vi "select energy_old.vi"(8 "Error In":errorcluster, 9 "List ROI in":dbl[][](array[numeric]), 10 "List Peak":string[][](table)=[["0", "0.738169", "8216.078017"], ["1", "1.925791", "11797.605609"], ["2", "2.296686", "59445.586632"], ["3", "2.951953", "7958.809520"], ["4", "3.301930", "5536.954047"], ["5", "3.693063", "592063.911968"], ["6", "4.012579", "88599.650063"], ["7", "5.456304", "6013.116723"], ["8", "5.905392", "7038.874622"], ["9", "6.404196", "22471.618393"], ["10", "7.049745", "8038.961303"], ["11", "7.336853", "5649.863203"], ["12", "7.978842", "3458.992769"], ["13", "8.617482", "7301.160509"], ["14", "9.554502", "1097.160220"], ["15", "10.523191", "20487.327187"], ["16", "11.054270", "2935.510385"], ["17", "11.234771", "2776.270069"], ["18", "12.573155", "28067.247871"], ["19", "13.048495", "7100.524309"], ["20", "13.060056", "7093.993228"], ["21", "13.100857", "7126.608473"], ["22", "13.283153", "7227.068614"], ["23", "14.060270", "10970.472713"], ["24", "14.659482", "8813.189447"], ["25", "15.701110", "4886.263831"], ["26", "16.589220", "151655.425908"], ["27", "17.295466", "73726.613413"], ["28", "18.547307", "16625.597400"], ["29", "19.386897", "11325.808412"], ["30", "23.791659", "1504.095156"], ["31", "24.239552", "1887.308691"], ["32", "24.942128", "13678.898904"]], 11 "Spectrum":cluster{"Channels":dbl[], "Intensity":dbl[]}[](graph)) -> (0 "Error Out":errorcluster, 1 "List ROI in out":dbl[][](array[numeric]), 2 "Peak Position":cluster{"Array":dbl[], "Array":dbl[]}, 3 "Elements":string[][](table))   [LabVIEW 2020]
uses:
  <vilib>/Utility/miscctls.llb/LVRowAndColumnTypeDef.ctl
  e287f4bb-419c-b64e-b283-fdec1ab58d66.vi
  8e2a2df9-f711-f049-943d-4995b6f05a7b.vi
  95577ca1-b70a-e540-a978-da85c0e4bb45.vi
  <vilib>/Utility/Data Type/Get Array Information.vi
  <vilib>/Utility/Data Type/Get Type Information.vi
panel:
  in  "Add":bool
  in  "ordinate":u16(ring) items=["Linear", "Logarithmic"]
  in  "doubt":bool
  in  "reset":bool
  out "List In":cluster{"Channels":dbl[], "Intensity":dbl[]}
  out "Data In":cluster{"Channels":dbl[], "Intensity":dbl[]}
  out "Element Position Peaks":dbl[][](array[numeric])
  out "Best Match":string[][](table)
  in  "exit":bool
  # "?"
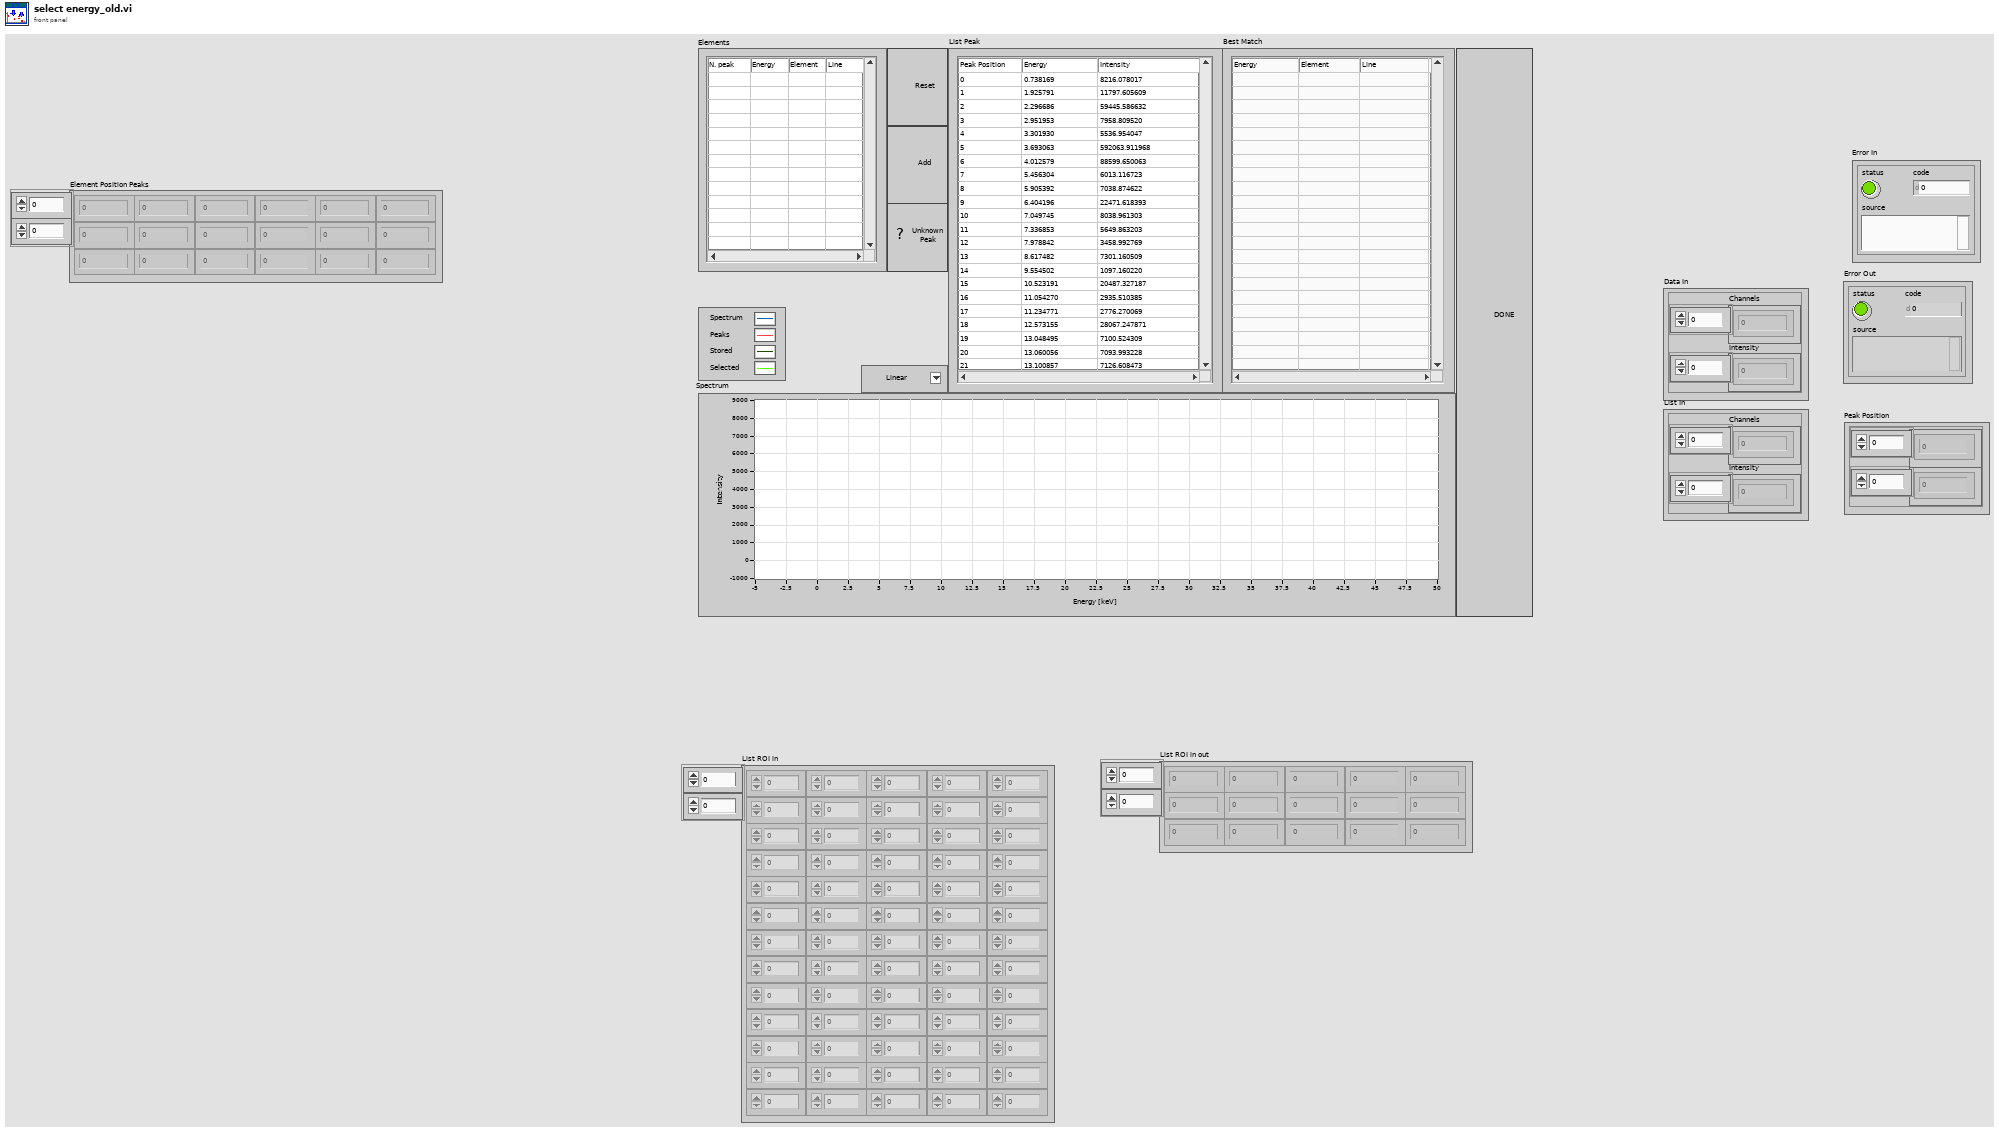
[diagram p1: front panel]
types:
  T1 = typedef "LVRowAndColumnTypeDef.ctl" = cluster{"Row":i32, "Column":i32}
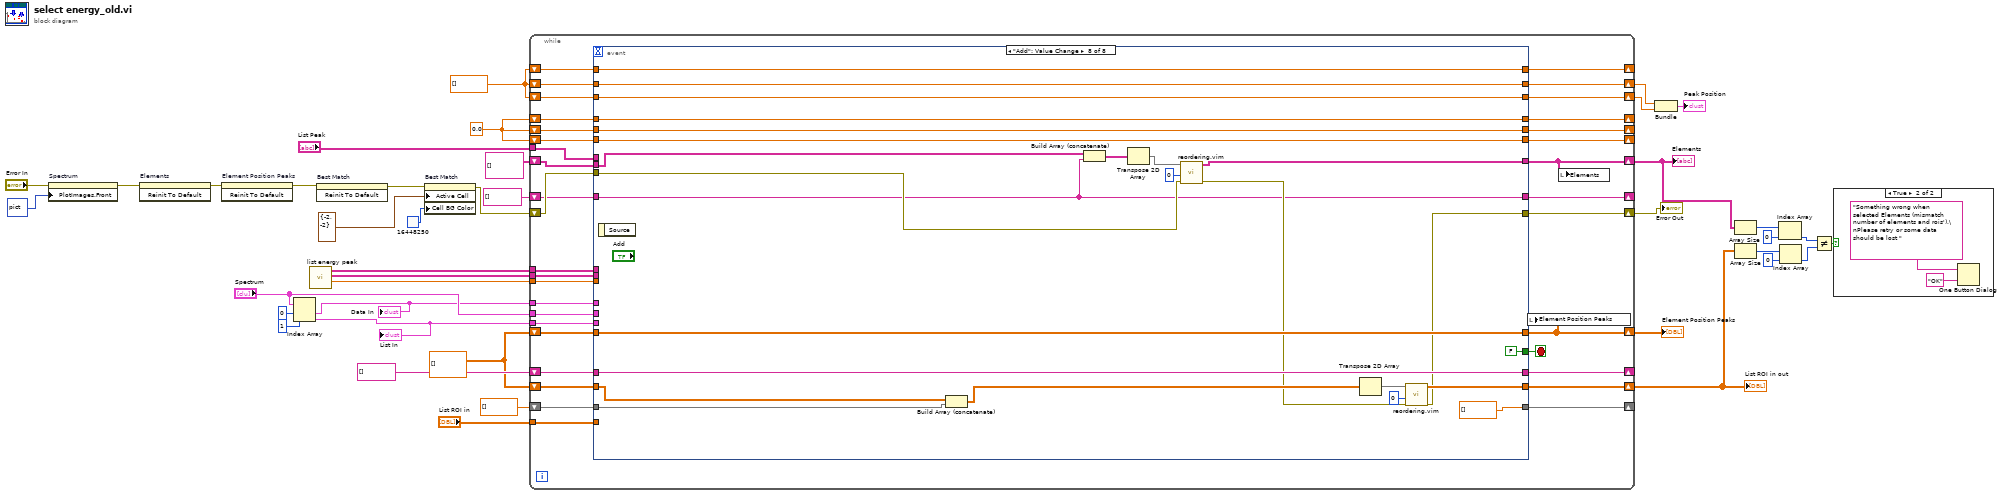
[diagram p0: block diagram]
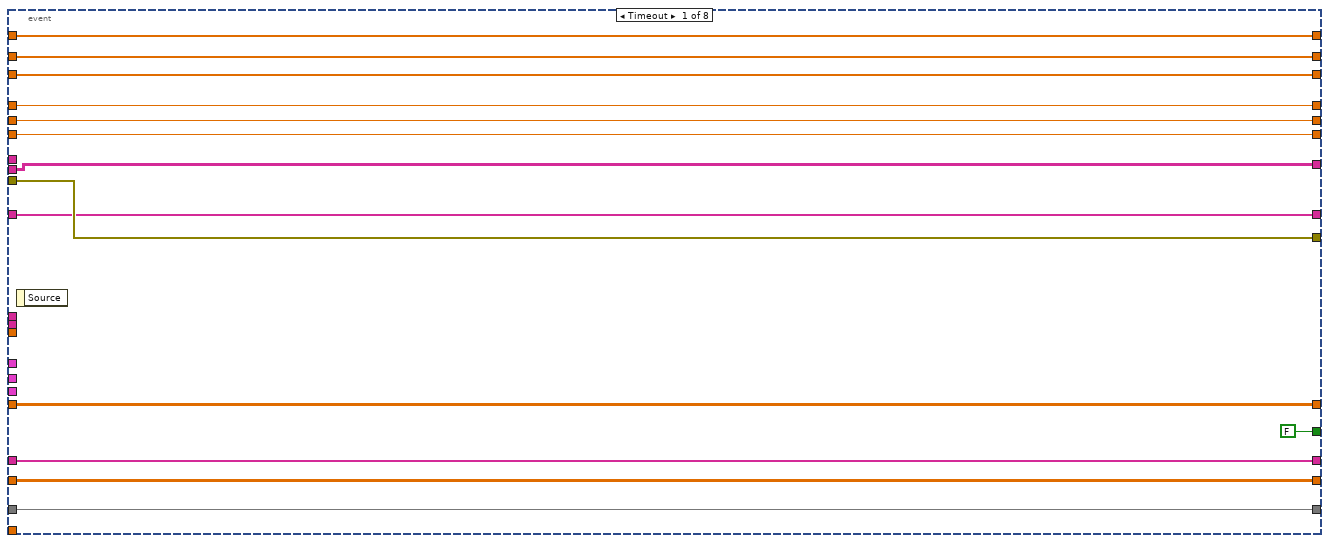
[diagram p3: hidden frame]
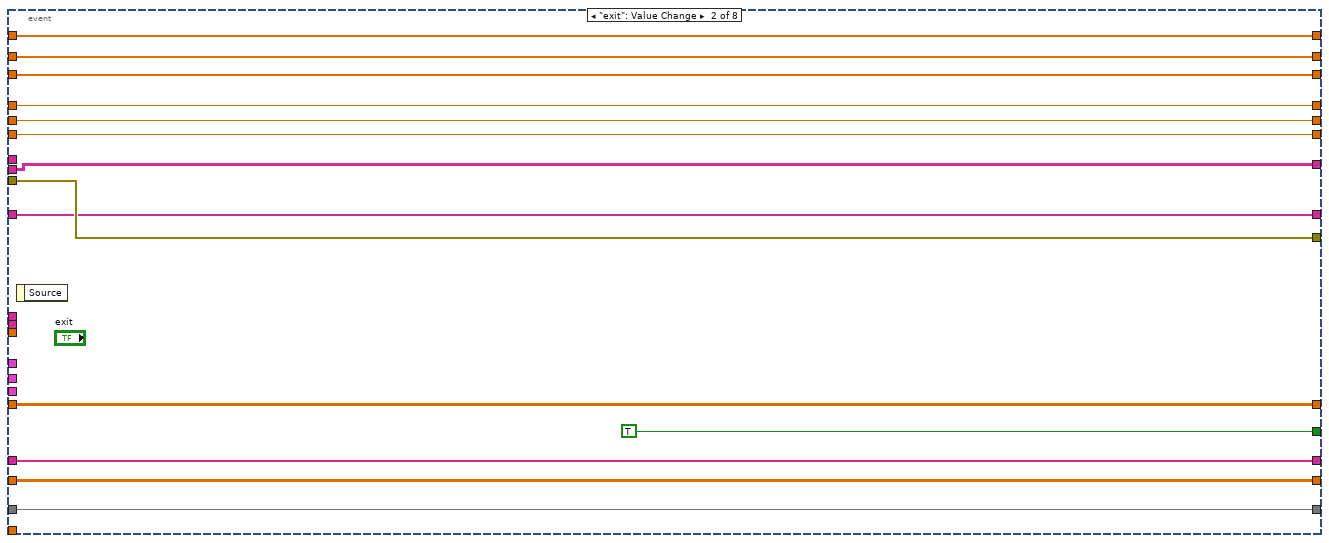
[diagram p4: hidden frame]
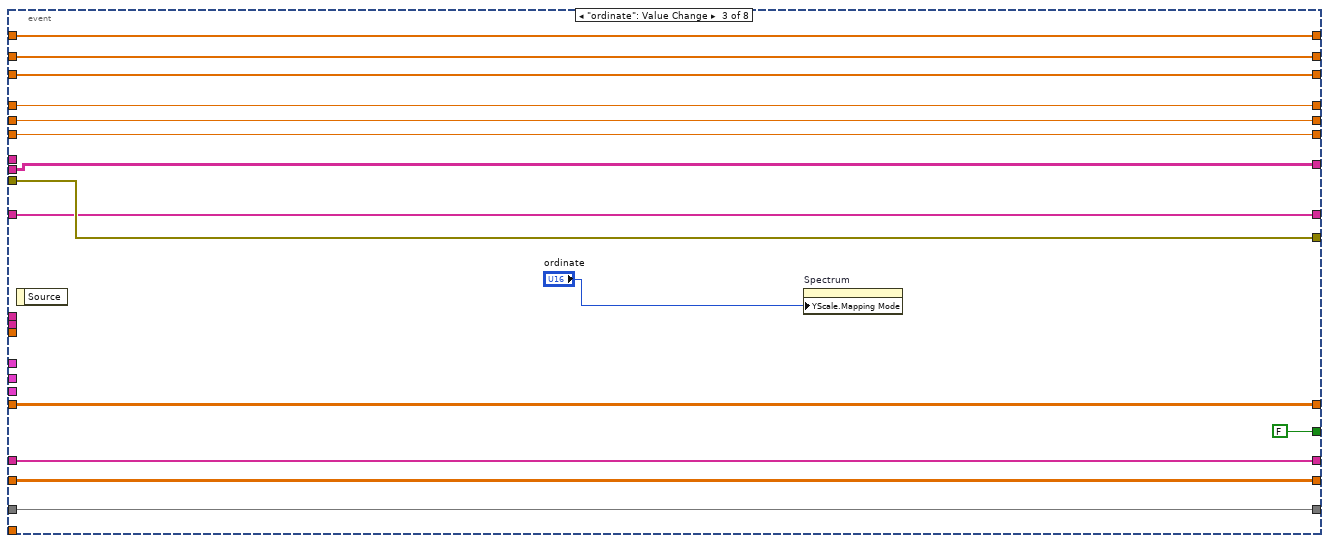
[diagram p5: hidden frame]
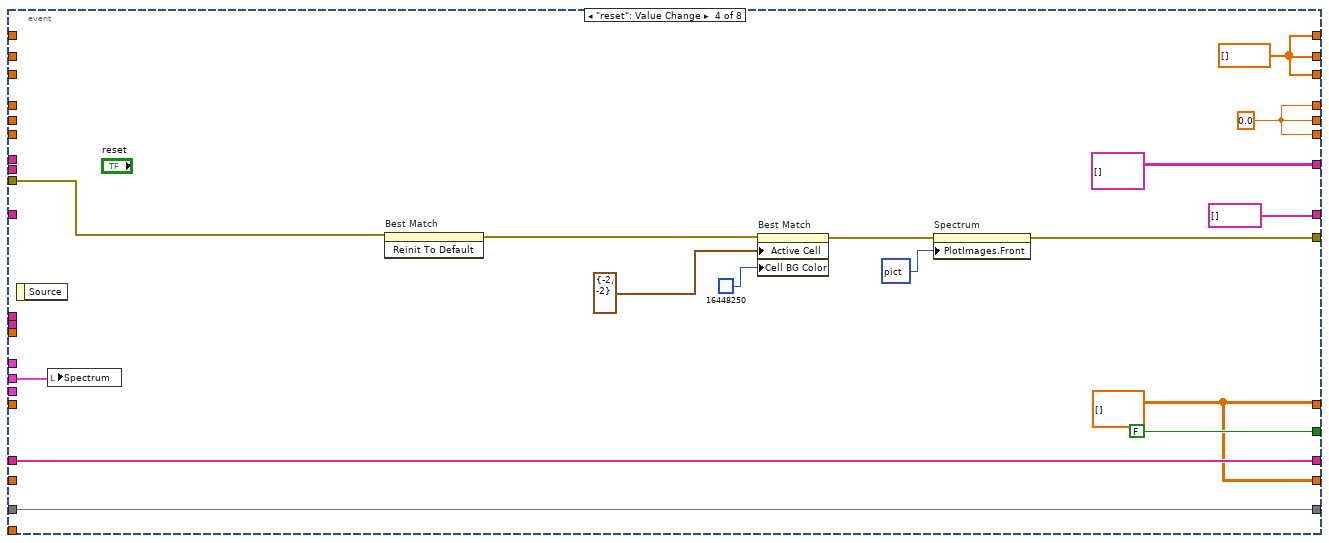
[diagram p6: hidden frame]
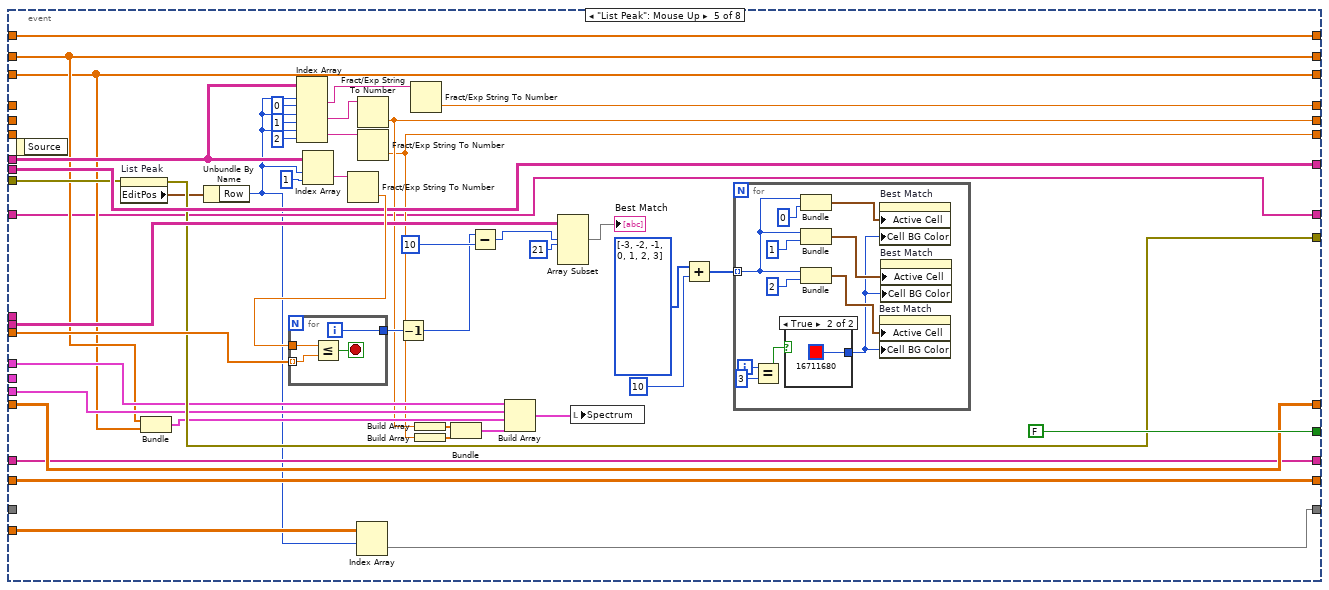
[diagram p7: hidden frame]
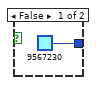
[diagram p8: hidden frame]
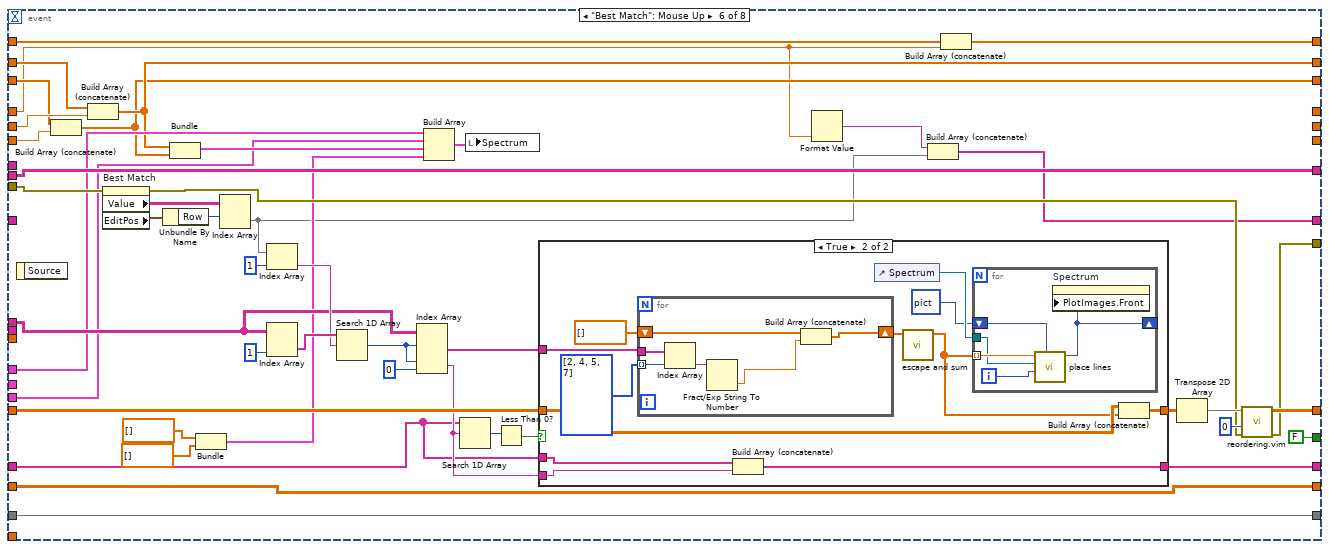
[diagram p9: hidden frame]
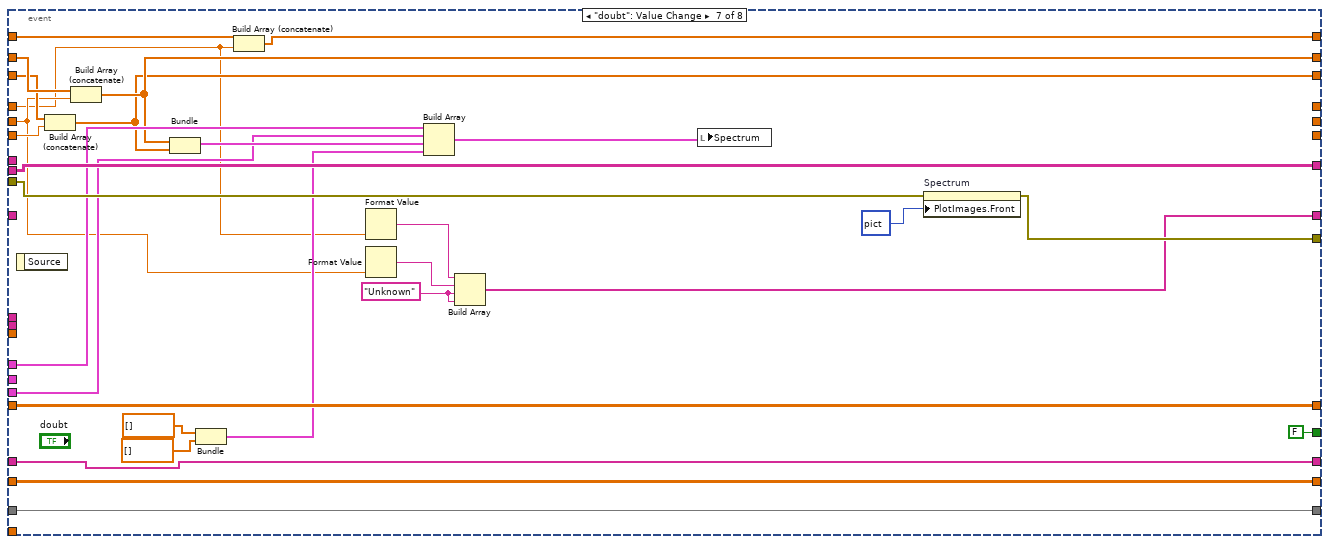
[diagram p11: hidden frame]
diagram:
  w2 = 0.0
  w1 = dbl[] []
  w13 = dbl[][] []
  n1 = property on="Spectrum" class="XYGraph (strict)"(error in="Error In", "PlotImages.Front"=picture data[5B] ("line to place")) -> (error out=w25:errorcluster)  [unwired: 1 in, 1 out]
  n2 = invoke on="Elements" class="Tbl (strict)" method="Reinit To Default"(error in=w25) -> (error out=w31:errorcluster)  [unwired: 2 in, 2 out]
  n3 = invoke on="Element Position Peaks" class="Arr (strict)" method="Reinit To Default"(error in=w31) -> (error out=w30:errorcluster)  [unwired: 2 in, 2 out]
  n4 = Index Array(array="Spectrum", index #1=0 ("index"), index #2=1 ("index")) -> (element #1=w20:cluster{"Channels":dbl[], "Intensity":dbl[]}, element #2=w19:cluster{"Channels":dbl[], "Intensity":dbl[]})
  "Data In" <- w20
  "List In" <- w19
  n5 = call "list energy peak.vi"() -> ("Energies Ordered"=w39:dbl[], "List Ordered"=w40:string[][], "List"=w34:string[][])  [unwired: 9 in]
  n6 = invoke on="Best Match" class="Tbl (strict)" method="Reinit To Default"(error in=w30) -> (error out=w37:errorcluster)  [unwired: 2 in, 2 out]
  n7 = property on="Best Match" class="Tbl (strict)"(error in=w37, "Active Cell"=T1 {"Row"=-2, "Column"=-2} ("Active Cell:Active Cell"), "Cell BG Color"=u32 16448250) -> (error out=w29:errorcluster)  [unwired: 1 in, 1 out]
  n8 = while {
    tunnel: "List Peak" -> [w75]
    tunnel: w40 -> [w72]
    tunnel: w39 -> [w74]
    tunnel: w34 -> [w71]
    shift-right: [w68] -> w7
    shift-left: string[][] [] -> [w70]
    shift-right: [w67] -> w32
    shift-left: w13 -> [w69]
    tunnel: "Spectrum" -> [w60]
    shift-right: [w66] -> w28
    shift-left: w29 -> [w65]
    shift-right: [w64] -> _
    shift-left: string[] [] -> [w63]
    shift-right: [w62] -> w17
    shift-left: w1 -> [w61]
    shift-right: [w59] -> w18
    shift-left: w1 -> [w58]
    tunnel: w20 -> [w57]
    tunnel: w19 -> [w56]
    shift-right: [w54] -> _
    shift-left: w2 -> [w52]
    shift-right: [w55] -> _
    shift-left: w2 -> [w53]
    shift-right: [w51] -> _
    shift-left: string[] [] ("Value") -> [w50]
    shift-right: [w49] -> w6
    shift-left: w13 -> [w48]
    tunnel: "List ROI in" -> [w47]
    shift-right: [w45] -> _
    shift-left: dbl[] [] -> [w46]
    shift-right: [w44] -> _
    shift-left: w2 -> [w43]
    shift-right: [w42] -> _
    shift-left: w1 -> [w41]
    stop <- w73 stop-if-true
    n9 = event shown="[7] \"Add\": Value Change" {
      selector: _ -> [_ _ _ _ _ _ _ _]
      dyn-events: _ -> [_ _ _ _ _ _ _ _]
      timeout: _ -> [_ _ _ _ _ _ _ _]
      tunnel: w75 -> [_ _ _ _ w159 _ _ _]
      tunnel: w74 -> [_ _ _ _ w177 _ _ _]
      tunnel: [FALSE ("Stop Button") TRUE ("Stop Button") FALSE ("Stop Button") FALSE ("Stop Button") FALSE ("Stop Button") FALSE ("Stop Button") FALSE ("Stop Button") FALSE ("Stop Button")] -> w73
      tunnel: w72 -> [_ _ _ _ w174 _ _ _]
      tunnel: w71 -> [_ _ _ _ _ w237 _ _]
      tunnel: [w88 w102 w117 string[][] [] ("Data Out") w165 w236 w298 w315] -> w68
      tunnel: w70 -> [w88 w102 w117 _ w165 w236 w298 w316]
      tunnel: [w87 w101 w116 w121 w164 w233 w297 w312] -> w67
      tunnel: w69 -> [w87 w101 w116 _ w164 w235 w297 w312]
      tunnel: [w86 w100 w115 w125 w162 w227 w280 w303] -> w66
      tunnel: w65 -> [w86 w100 w115 w129 w163 w229 w295 w314]
      tunnel: [w85 w99 w114 w128 w161 w221 w282 w311] -> w64
      tunnel: w63 -> [w85 w99 w114 w128 w161 w220 w282 w311]
      tunnel: [w84 w97 w112 w119 w150 w207 w283 w322] -> w62
      tunnel: w61 -> [w84 w97 w112 _ w150 w209 w285 w322]
      tunnel: w60 -> [_ _ _ w124 _ _ _ _]
      tunnel: [w83 w98 w113 w119 w151 w210 w286 w323] -> w59
      tunnel: w58 -> [w83 w98 w113 _ w151 w212 w287 w323]
      tunnel: w57 -> [_ _ _ _ w153 w217 w292 _]
      tunnel: w56 -> [_ _ _ _ w152 w216 w291 _]
      tunnel: [w82 w96 w111 w120 w145 _ _ w321] -> w55
      tunnel: [w81 w95 w110 w120 w144 _ _ w320] -> w54
      tunnel: w53 -> [w82 w96 w111 _ _ w211 w273 w321]
      tunnel: w52 -> [w81 w95 w110 _ _ w208 w284 w320]
      tunnel: [w80 w94 w108 string[] [] ("Value") w143 w199 w277 w299] -> w51
      tunnel: w50 -> [w80 w94 w108 _ w143 _ _ w299]
      tunnel: [w79 w93 w107 w121 w142 w204 w275 w305] -> w49
      tunnel: w48 -> [w79 w93 w107 _ w142 w204 w275 w310]
      tunnel: w47 -> [_ _ _ _ w141 _ _ _]
      tunnel: w46 -> [w78 w92 w106 w122 _ w205 w276 w309]
      tunnel: [w78 w92 w106 w122 w140 w205 w276 dbl[] []] -> w45
      tunnel: [w77 w91 w105 w120 w136 _ _ w301] -> w44
      tunnel: w43 -> [w77 w91 w105 _ _ w201 w270 w301]
      tunnel: [w76 w90 w104 w119 w135 w202 w272 w300] -> w42
      tunnel: w41 -> [w76 w90 w104 _ w135 w203 w274 w300]
      event Timeout {
        n10 = event-data() -> ()  [unwired: 1 in, 1 out]
      }
      event "exit": Value Change {
        n11 = event-data() -> ()  [unwired: 1 in, 1 out]
      }
      event "ordinate": Value Change {
        n12 = event-data() -> ()  [unwired: 1 in, 1 out]
        n13 = property on="Spectrum" class="XYGraph (strict)"("YScale.Mapping Mode"="ordinate") -> ()  [unwired: 2 in, 2 out]
      }
      event "reset": Value Change {
        w120 = 0.0
        w119 = dbl[] []
        w121 = dbl[][] [] ("Data Out")
        n14 = event-data() -> ()  [unwired: 1 in, 1 out]
        n15 = local write "Spectrum"(w124) -> ()
        n16 = invoke on="Best Match" class="Tbl (strict)" method="Reinit To Default"(error in=w129) -> (error out=w134:errorcluster)  [unwired: 2 in, 2 out]
        n17 = property on="Best Match" class="Tbl (strict)"(error in=w134, "Active Cell"=T1 {"Row"=-2, "Column"=-2} ("Active Cell:Active Cell"), "Cell BG Color"=u32 16448250) -> (error out=w126:errorcluster)  [unwired: 1 in, 1 out]
        n18 = property on="Spectrum" class="XYGraph (strict)"(error in=w126, "PlotImages.Front"=picture data[5B] ("line to place")) -> (error out=w125:errorcluster)  [unwired: 1 in, 1 out]
      }
      event "List Peak": Mouse Up {
        n19 = event-data() -> ()  [unwired: 1 in, 1 out]
        n20 = property on="List Peak" class="Tbl (strict)"(error in=w163) -> (error out=w162:errorcluster, "EditPos"=w160:T1)  [unwired: 1 in, 1 out]
        n21 = Bundle(w151, w150) -> (w149:cluster{dbl[], dbl[]})  [unwired: 1 in]
        n22 = Unbundle By Name(w160) -> ("Row"=w139:i32)
        n23 = Index Array(array=w159, index (row) #1=w139, index (col) #1=0 ("disabled index (col)"), index (row) #2=w139, index (col) #2=1 ("disabled index (col)"), index (row) #3=w139, index (col) #3=2 ("disabled index (col)")) -> (element #1=w137:string, element #2=w156:string, element #3=w155:string)
        n24 = Index Array(array=w159, index (row)=w139, index (col)=1 ("disabled index (col)")) -> (element=w179:string)
        n25 = Fract/Exp String To Number(string=w179) -> (number=w178:dbl)  [unwired: 3 in, 1 out]
        n26 = for {
          tunnel: w178 -> [w197]
          tunnel: w177 -> [w196] mode=indexing
          tunnel: [w194] -> w175
          i -> [w194]
          stop <- w195 stop-if-true
          n27 = Less Or Equal?(x=w197, y=w196) -> (x <= y?=w195:bool)
        }
        n28 = Index Array(array=w141, index (row)=w139) -> (element=w140:dbl[])  [unwired: 1 in]
        n29 = Fract/Exp String To Number(string=w156) -> (number=w145:dbl)  [unwired: 3 in, 1 out]
        n30 = Fract/Exp String To Number(string=w155) -> (number=w144:dbl)  [unwired: 3 in, 1 out]
        n31 = Decrement(x=w175) -> (x-1=w168:i32)
        n32 = Fract/Exp String To Number(string=w137) -> (number=w136:dbl)  [unwired: 3 in, 1 out]
        n33 = Build Array(w145) -> (w147:dbl[])
        n34 = Build Array(w144) -> (w146:dbl[])
        n35 = Bundle(w147, w146) -> (w148:cluster{dbl[], dbl[]})  [unwired: 1 in]
        n36 = Subtract(x=w168, y=10) -> (x-y=w171:i32)
        n37 = Build Array(w153, w152, w149, w148) -> (w154:cluster{"Channels":dbl[], "Intensity":dbl[]}[])
        n38 = Array Subset(array=w174, index (row)=w171, length (row)=21 ("length")) -> (→"Best Match":string[][])  [unwired: 2 in]
        n39 = local write "Spectrum"(w154) -> ()
        n40 = Add(x=i32[] [-3, -2, -1, 0, 1, 2, 3], y=10) -> (x+y=w167:i32[])
        n41 = for {
          tunnel: w167 -> [w183] mode=indexing
          i -> [w191]
          n42 = Equal?(x=w191, y=3) -> (x = y?=w189:bool)
          n43 = case shown="True" w189 {
            tunnel: [u32 9567230 u32 16711680] -> w181
            frame False {
            }
            frame True {
            }
          }
          n44 = Bundle(w183, 0) -> (w182:cluster{i32, i32})  [unwired: 1 in]
          n45 = Bundle(w183, 1) -> (w186:cluster{i32, i32})  [unwired: 1 in]
          n46 = Bundle(w183, 2) -> (w185:cluster{i32, i32})  [unwired: 1 in]
          n47 = property on="Best Match" class="Tbl (strict)"("Active Cell"=w182, "Cell BG Color"=w181) -> ()  [unwired: 2 in, 2 out]
          n48 = property on="Best Match" class="Tbl (strict)"("Active Cell"=w185, "Cell BG Color"=w181) -> ()  [unwired: 2 in, 2 out]
          n49 = property on="Best Match" class="Tbl (strict)"("Active Cell"=w186, "Cell BG Color"=w181) -> ()  [unwired: 2 in, 2 out]
        }
      }
      event "Best Match": Mouse Up {
        n50 = event-data() -> ()  [unwired: 1 in, 1 out]
        n51 = Build Array (concatenate)(w209, w208) -> (w207:dbl[])
        n52 = Build Array (concatenate)(w212, w211) -> (w210:dbl[])
        n53 = property on="Best Match" class="Tbl (strict)"(error in=w229) -> (error out=w228:errorcluster, "Value"=w243:string[][], "EditPos"=w244:T1)  [unwired: 1 in, 1 out]
        n54 = Unbundle By Name(w244) -> ("Row"=w206:i32)
        n55 = Bundle(w210, w207) -> (w218:cluster{dbl[], dbl[]})  [unwired: 1 in]
        n56 = Bundle(dbl[] [], dbl[] []) -> (w213:cluster{dbl[], dbl[]})  [unwired: 1 in]
        n57 = Index Array(array=w243, index (row)=w206) -> (element=w200:string[])  [unwired: 1 in]
        n58 = Index Array(array=w200, index=1) -> (element=w239:string)
        n59 = Index Array(array=w237, index (col)=1 ("disabled index (col)")) -> (element=w240:string[])  [unwired: 1 in]
        n60 = Search 1D Array(1D array=w240, element=w239) -> (index of element=w226:i32)  [unwired: 1 in]
        n61 = Index Array(array=w237, index (row) #1=w226, index (row) #2=w226, index (col) #2=0 ("disabled index (col)")) -> (element #1=w238:string[], element #2=w222:string)  [unwired: 1 in]
        n62 = Build Array(w217, w216, w218, w213) -> (w219:cluster{"Channels":dbl[], "Intensity":dbl[]}[])
        n63 = Search 1D Array(1D array=w220, element=w222) -> (index of element=w224:i32)  [unwired: 1 in]
        n64 = local write "Spectrum"(w219) -> ()
        n65 = Less Than 0?(x=w224) -> (x < 0?=w223:bool)
        n66 = case shown="True" w223 {
          tunnel: w238 -> [_ w258]
          tunnel: w235 -> [w246 w255]
          tunnel: [w246 w254] -> w232
          tunnel: w222 -> [_ w252]
          tunnel: [w245 w251] -> w221
          tunnel: w220 -> [w245 w250]
          frame False {
          }
          frame True {
            n67 = for {
              tunnel: w258 -> [w269]
              tunnel: i32[] [2, 4, 5, 7] -> [w268] mode=indexing
              shift-right: [w267] -> w253
              shift-left: dbl[] [] -> [w266]
              n68 = Index Array(array=w269, index=w268) -> (element=w265:string)
              n69 = Fract/Exp String To Number(string=w265) -> (number=w264:dbl)  [unwired: 3 in, 1 out]
              n70 = Build Array (concatenate)(w266, w264) -> (w267:dbl[])
            }
            n71 = Build Array (concatenate)(w250, w252) -> (w251:string[])
            n72 = control-ref of="Spectrum"() -> (w248:refnum<vi>)
            n73 = call "escape and sum.vi"("List in"=w253) -> ("List Out"=w249:dbl[])  [unwired: 10 in]
            n74 = for {
              tunnel: w249 -> [w263] mode=indexing
              tunnel: w248 -> [w261]
              shift-right: [w260] -> _
              shift-left: picture data[5B] ("line to place") -> [w259]
              i -> [w262]
              n75 = call "place lines.vi"("picture in"=w259, "line"=w262, "Graph"=w261, "Energy"=w263) -> ("line to place"=w260:picture)  [unwired: 7 in]
              n76 = property on="Spectrum" class="XYGraph (strict)"("PlotImages.Front"=w260) -> ()  [unwired: 2 in, 2 out]
            }
            n77 = Build Array (concatenate)(w255, w249) -> (w254:dbl[][])
          }
        }
        n78 = Format Value(value (0)=w201) -> (output string=w198:string)  [unwired: 2 in]
        n79 = Build Array (concatenate)(w198, w200) -> (w199:string[])
        n80 = Build Array (concatenate)(w203, w201) -> (w202:dbl[])
        n81 = Transpose 2D Array(2D array=w232) -> (transposed array=w231:dbl[][])
        n82 = call "reordering.vim"("error in (no error)"=w228, "Row to Reorder"=0, "Data In"=w231) -> ("Error Out"=w227:errorcluster, "Data Out"=w233:dbl[][])  [unwired: 7 in]
      }
      event "doubt": Value Change {
        w279 = "Unknown"
        n83 = event-data() -> ()  [unwired: 1 in, 1 out]
        n84 = Build Array (concatenate)(w285, w284) -> (w283:dbl[])
        n85 = Build Array (concatenate)(w287, w273) -> (w286:dbl[])
        n86 = Bundle(w286, w283) -> (w293:cluster{dbl[], dbl[]})  [unwired: 1 in]
        n87 = Bundle(dbl[] [], dbl[] []) -> (w288:cluster{dbl[], dbl[]})  [unwired: 1 in]
        n88 = Build Array (concatenate)(w274, w270) -> (w272:dbl[])
        n89 = Format Value(value (0)=w270) -> (output string=w271:string)  [unwired: 2 in]
        n90 = Format Value(value (0)=w273) -> (output string=w278:string)  [unwired: 2 in]
        n91 = Build Array(w292, w291, w293, w288) -> (w294:cluster{"Channels":dbl[], "Intensity":dbl[]}[])
        n92 = Build Array(w271, w278, w279, w279) -> (w277:string[])
        n93 = local write "Spectrum"(w294) -> ()
        n94 = property on="Spectrum" class="XYGraph (strict)"(error in=w295, "PlotImages.Front"=picture data[5B] ("line to place")) -> (error out=w280:errorcluster)  [unwired: 1 in, 1 out]
      }
      event "Add": Value Change {
        n95 = event-data() -> ()  [unwired: 1 in, 1 out]
        n96 = Build Array (concatenate)(w310, w309) -> (w306:dbl[][])
        n97 = Build Array (concatenate)(w316, w299) -> (w319:string[][])
        n98 = Transpose 2D Array(2D array=w319) -> (transposed array=w318:string[][])
        n99 = call "reordering.vim"("error in (no error)"=w314, "Row to Reorder"=0, "Data In"=w318) -> ("Error Out"=w304:errorcluster, "Data Out"=w315:string[][])  [unwired: 7 in]
        n100 = Transpose 2D Array(2D array=w306) -> (transposed array=w307:dbl[][])
        n101 = call "reordering.vim"("error in (no error)"=w304, "Row to Reorder"=0, "Data In"=w307) -> ("Error Out"=w303:errorcluster, "Data Out"=w305:dbl[][])  [unwired: 7 in]
      }
    }
    n102 = local write "Element Position Peaks"(w67) -> ()
    n103 = local write "Elements"(w68) -> ()
  }
  "Element Position Peaks" <- w32
  "Elements" <- w7
  "Error Out" <- w28
  "List ROI in out" <- w6
  n104 = Bundle(w18, w17) -> (→"Peak Position":cluster{dbl[], dbl[]})  [unwired: 1 in]
  n105 = Array Size(array=w7) -> (size(s)=w11:i32[])
  n106 = Array Size(array=w6) -> (size(s)=w9:i32[])
  n107 = Index Array(array=w11, index=0) -> (element=w4:i32)
  n108 = Index Array(array=w9, index=0) -> (element=w5:i32)
  n109 = Not Equal?(x=w4, y=w5) -> (x != y?=w3:bool)
  n110 = case shown="True" w3 {
    frame False {
    }
    frame True {
      n111 = One Button Dialog(message="Something wrong when selected Elements (mismatch number of elements and rois').\nPlease retry or some data should be lost ", button name ("OK")="OK") -> ()  [unwired: 1 out]
    }
  }
